vi "Engine - Script RT Driver For Runtime Configuration.vi"(8 "error in":errorcluster, 10 "Support Runtime Configuration":bool, 11 "RT Driver VI Path":path) -> (0 "error out":errorcluster)   [LabVIEW 2020, in "NIVS_Consolidated_CDW_MetaDataObj.lvclass"]
uses:
  NIVS_Consolidated_CDW_MetaDataObj.lvclass
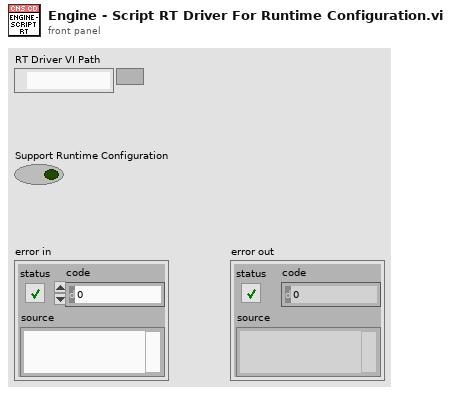
[diagram p1: front panel]
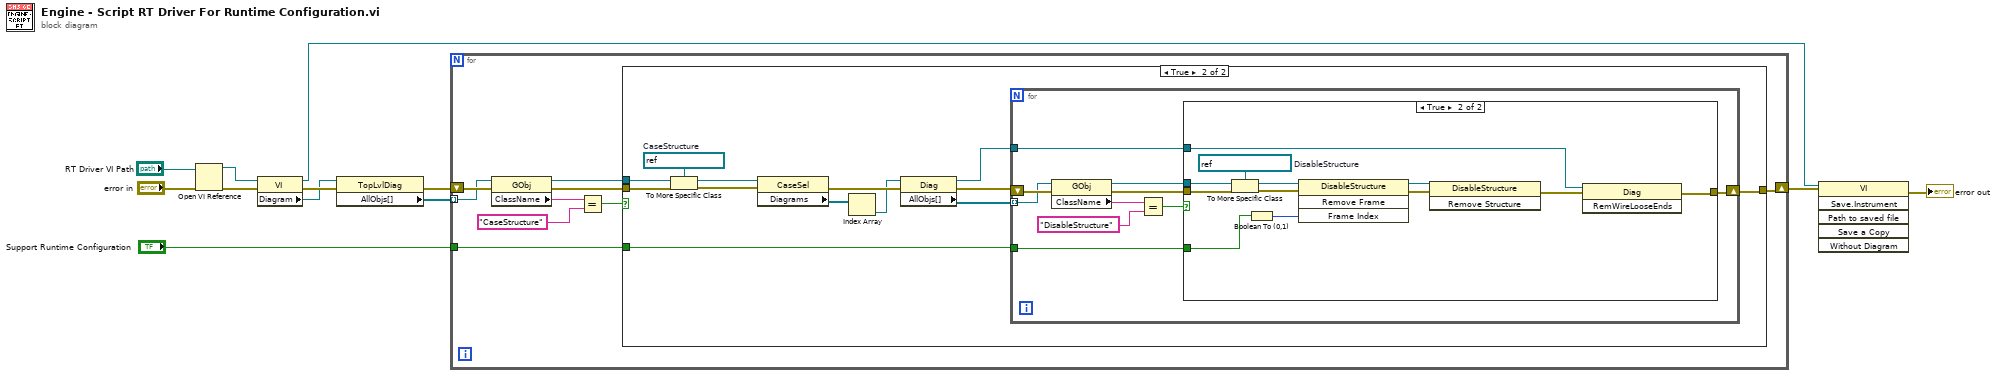
[diagram p0: block diagram]
diagram:
  n1 = Open VI Reference(vi path="RT Driver VI Path", error in (no error)="error in") -> (vi reference=w6:refnum<vi>, error out=w12:errorcluster)  [unwired: 4 in]
  n2 = property class="VI"(reference=w6, error in=w12) -> (reference out=w1:refnum<vi>, error out=w11:errorcluster, "Diagram"=w5:refnum<vi>)
  n3 = property class="TopLvlDiag"(reference=w5, error in=w11) -> (error out=w10:errorcluster, "AllObjs[]"=w4:refnum<vi>[])  [unwired: 1 out]
  n4 = for {
    shift-right: [w19] -> w8
    shift-left: w10 -> [w21]
    tunnel: w4 -> [w18] mode=indexing
    tunnel: "Support Runtime Configuration" -> [w13]
    n5 = property class="GObj"(reference=w18, error in=w21) -> (reference out=w14:refnum<vi>, error out=w20:errorcluster, "ClassName"=w17:string)
    n6 = Equal?(x=w17, y="CaseStructure") -> (x = y?=w15:bool)
    n7 = case shown="True" w15 {
      tunnel: w14 -> [_ w30]
      tunnel: w13 -> [_ w23]
      tunnel: w20 -> [w22 w35]
      tunnel: [w22 w31] -> w19
      frame False {
      }
      frame True {
        w29 = refnum<vi> refnum  # CaseStructure
        n8 = To More Specific Class(target class=w29, reference=w30, error in=w35) -> (specific class reference=w28:refnum<vi>, error out=w34:errorcluster)
        n9 = property class="CaseSel"(reference=w28, error in=w34) -> (error out=w33:errorcluster, "Diagrams"=w27:refnum<vi>[])  [unwired: 1 out]
        n10 = Index Array(array=w27) -> (element=w26:refnum<vi>)  [unwired: 1 in]
        n11 = property class="Diag"(reference=w26, error in=w33) -> (reference out=w25:refnum<vi>, error out=w32:errorcluster, "AllObjs[]"=w24:refnum<vi>[])
        n12 = for {
          shift-right: [w43] -> w31
          shift-left: w32 -> [w45]
          tunnel: w24 -> [w42] mode=indexing
          tunnel: w23 -> [w37]
          tunnel: w25 -> [w36]
          n13 = property class="GObj"(reference=w42, error in=w45) -> (reference out=w38:refnum<vi>, error out=w44:errorcluster, "ClassName"=w41:string)
          n14 = Equal?(x=w41, y="DisableStructure") -> (x = y?=w39:bool)
          n15 = case shown="True" w39 {
            tunnel: w38 -> [_ w53]
            tunnel: w37 -> [_ w48]
            tunnel: w44 -> [w46 w58]
            tunnel: [w46 w55] -> w43
            tunnel: w36 -> [_ w47]
            frame False {
            }
            frame True {
              w52 = refnum<vi> refnum  # DisableStructure
              n16 = To More Specific Class(target class=w52, reference=w53, error in=w58) -> (specific class reference=w51:refnum<vi>, error out=w54:errorcluster)
              n17 = Boolean To (0,1)(Boolean=w48) -> (0, 1=w50:i16)
              n18 = invoke class="DisableStructure" method="Remove Frame"(reference=w51, error in=w54, "Frame Index"=w50) -> (reference out=w49:refnum<vi>, error out=w57:errorcluster)  [unwired: 1 in, 2 out]
              n19 = invoke class="DisableStructure" method="Remove Structure"(reference=w49, error in=w57) -> (error out=w56:errorcluster)  [unwired: 1 in, 2 out]
              n20 = invoke class="Diag" method="RemWireLooseEnds"(reference=w47, error in=w56) -> (error out=w55:errorcluster)  [unwired: 1 in, 2 out]
            }
          }
        }
      }
    }
  }
  n21 = invoke class="VI" method="Save.Instrument"(reference=w1, error in=w8) -> (error out=→"error out":errorcluster)  [unwired: 4 in, 5 out]
